vi "XPS lauch async read.vi"(8 "error in (no error)":errorcluster, 11 "NewportXPS.lvclass":refnum<class "NewportXPS.lvclass">) -> (0 "error out":errorcluster, 2 "Acq Data out":T1, 3 "NewportXPS.lvclass out":refnum<class "NewportXPS.lvclass">)   [LabVIEW 2020, in "NewportXPS.lvclass"]
uses:
  NewportXPS.lvclass
  XPS Acquire FGV.ctl
  shared/stop FGV control.ctl
  XPS hardware acquire.vi
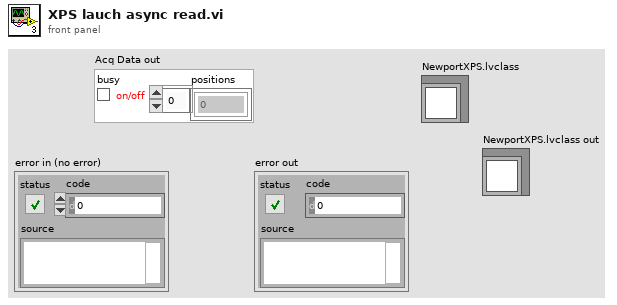
[diagram p1: front panel]
types:
  T1 = typedef "XPS Acquire FGV.ctl" = cluster{"busy":bool, "positions":dbl[]}
  T2 = typedef "stop FGV control.ctl" = enum16{"Clear", "Write", "Read"}
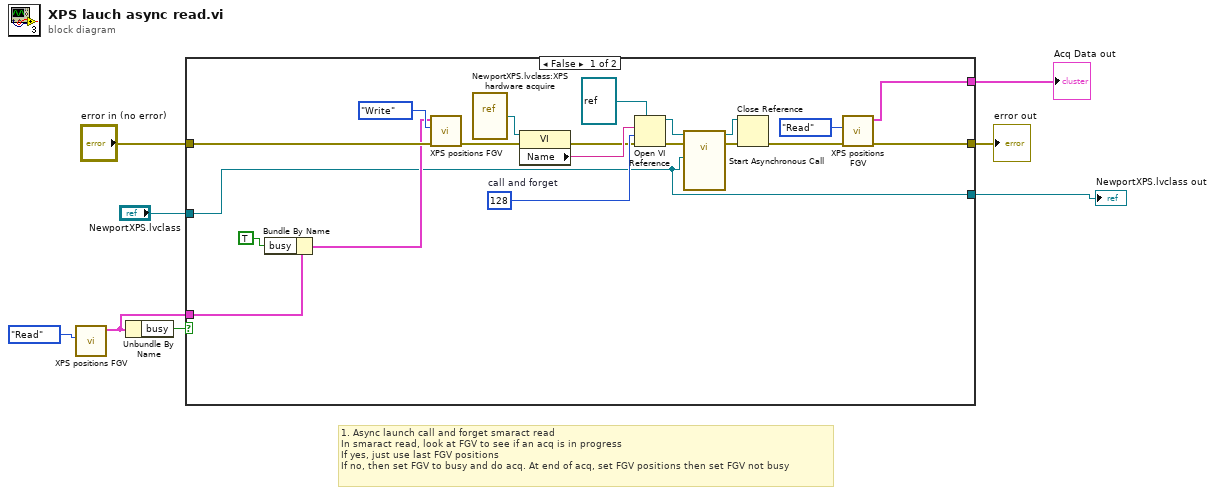
[diagram p0: block diagram]
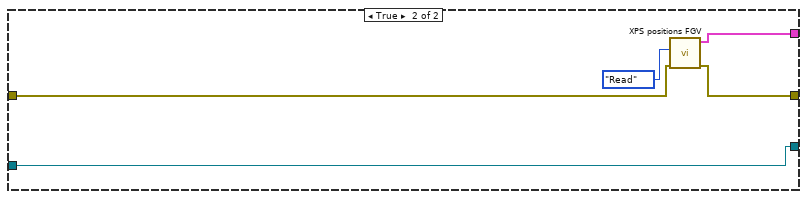
[diagram p2: hidden frame]
diagram:
  # "1. Async launch call and forget smaract read\nIn smaract read, look at FGV to see if an acq is in progress\nIf yes, just use last FGV positions\nIf no, then set FGV to busy and do acq. At end of acq, set FGV positions then set FGV not busy"
  n1 = call "XPS positions FGV.vi"("Function"=stop_FGV_control."Read") -> ("Acq Data out"=w4:T1)  [unwired: 9 in, 1 out]
  n2 = Unbundle By Name(w4) -> ("busy"=w6:bool)
  n3 = case shown="False" w6 {
    tunnel: [w9 w33] -> w2
    tunnel: [w12 w29] -> w8
    tunnel: "NewportXPS.lvclass" -> [w9 w33]
    tunnel: "error in (no error)" -> [w16 w31]
    tunnel: w4 -> [w18 _]
    tunnel: [w10 w30] -> w1
    frame False {
      w28 = 128  # call and forget
      n4 = Bundle By Name(cluster=w18, "busy"=TRUE) -> (w11:T1)
      n5 = call "XPS positions FGV.vi"("error in"=w16, "Function"=stop_FGV_control."Write", "Acq Data in"=w11) -> ("error out"=w15:errorcluster)  [unwired: 7 in, 1 out]
      n6 = vi-ref "NewportXPS.lvclass:XPS hardware acquire.vi"() -> (w20:refnum<vi>)
      n7 = property class="VI"(reference=w20, error in=w15) -> (error out=w21:errorcluster, "Name"=w22:string)  [unwired: 1 out]
      n8 = Open VI Reference(type specifier VI Refnum (for type only)=refnum<vi> refnum, vi path=w22, options=w28, error in (no error)=w21) -> (vi reference=w26:refnum<vi>, error out=w25:errorcluster)  [unwired: 2 in]
      n9 = call-by-ref "Start Asynchronous Call"(reference=w26, error in=w25, "Object in"=w9) -> (reference out=w23:refnum<vi>, error out=w24:errorcluster)  [unwired: 9 in, 2 out]
      n10 = Close Reference(reference=w23, error in (no error)=w24) -> (error out=w13:errorcluster)
      n11 = call "XPS positions FGV.vi"("error in"=w13, "Function"=stop_FGV_control."Read") -> ("error out"=w12:errorcluster, "Acq Data out"=w10:T1)  [unwired: 8 in]
    }
    frame True {
      n12 = call "XPS positions FGV.vi"("error in"=w31, "Function"=stop_FGV_control."Read") -> ("error out"=w29:errorcluster, "Acq Data out"=w30:T1)  [unwired: 8 in]
    }
  }
  "error out" <- w8
  "NewportXPS.lvclass out" <- w2
  "Acq Data out" <- w1
